vi "Handle MB Commands.vi"(4 "SP_CHAMBER":dbl, 6 "SP_DUT":dbl, 8 "error in (no error)":errorcluster, 10 "CMD REG":T1, 11 "Stand in":refnum<class "Stand.lvclass">) -> (0 "error out":errorcluster, 3 "Stand out":refnum<class "Stand.lvclass">)   [LabVIEW 2019, in "Stand.lvclass"]
uses:
  Stand.lvclass
  D:/GIT H4000/H4000/src/Device_class/Device.lvclass
  Modbus_class/CMD REG.ctl
  Stand.lvclass/Stand.ctl
  TypeDef/Mode.ctl
  Valve DIR.ctl
  Device_class/Device.lvclass/Device.ctl
  TypeDef/Direction.ctl
  TypeDef/State 44-1-2.ctl
  Valve Mode.ctl
  Device_class/GetFPGA.vi
  DoValve.vi
  Valve State Mode.vi
  DoValve.vi/e7d2c9dc-ba67-4685-b926-bcce34aa2778.vi
  DoValve.vi/628819af-fd07-4303-9780-3ddd467101db.vi
  Valve State Mode.vi/810e184e-eeb6-4027-a8ae-1422f3ce3d45.vi
  Valve State Mode.vi/57bd4a65-f3dc-44f5-8d68-677c2a197570.vi
  Valve State Mode.vi/03b2f9e4-fceb-4725-9b90-3fd10082a088.vi
  Valve State Mode.vi/2785bab5-dd59-4d13-b638-b9157202fa4a.vi
  Valve State Mode.vi/50faa4b8-a9b4-4cc6-ab66-55c42b424fcd.vi
  Valve State Mode.vi/c882c3fe-b7a7-4419-8f9b-6788aa23338b.vi
  Valve State Mode.vi/3d0d09bd-48e8-482f-b1e2-a36b2bb65234.vi
  Valve State Mode.vi/33d3f26a-dc4a-4f56-bf0a-61d04c5d7434.vi
  Valve State Mode.vi/52af9d47-24d1-4057-80bf-8d93bfb3d17d.vi
  Valve State Mode.vi/bbc9916c-129f-4456-975e-9c3ae3d5db66.vi
  Valve State Mode.vi/a6106d78-2bf9-477e-b655-d47fad07ddfe.vi
  Valve State Mode.vi/e2916439-03c6-4471-bb40-42242a636e27.vi
  Valve State Mode.vi/094228cb-a119-423c-9af8-5a16f059a318.vi
  Valve State Mode.vi/bf5ad1e6-a0ae-4579-ad74-ca8f304cb7cf.vi
  Valve State Mode.vi/eb4d2b76-f0f0-4e1d-bda0-609c5f37b4e7.vi
  Const All Valve.vi
  FPGA_API_class/FPGA API.lvclass
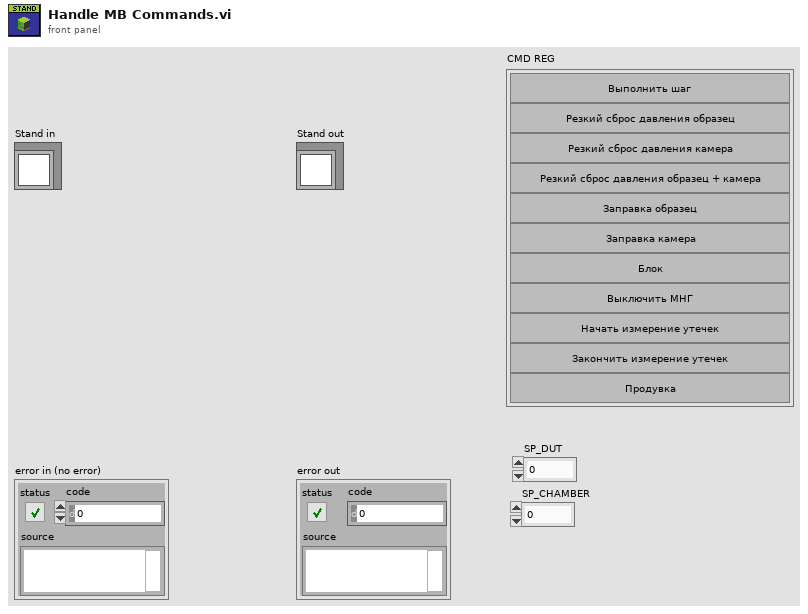
[diagram p1: front panel]
types:
  T1 = typedef "CMD REG.ctl" = cluster{"EXECUTE_SP":bool, "ALARM_PRESS_DOWN_DUT":bool, "ALARM_PRESS_DOWN_CHAMBER":bool, "ALARM_PRESS_DOWN_DUT_CHAMBER":bool, "FILING_DUT":bool, "FILING_CHAMBER":bool, "BLOCK":bool, "PUMP_STATION_OFF":bool, "Leak start":bool, "Leak stop":bool, "Drain":bool}
  T2 = typedef "Valve DIR.ctl" = enum16{"Air Valves: Open (DUT Filling)", "Air Valves: Open (Chamber Filling)", "Air Valves: Open (Pump Pressure DUT)", "Air Valves: Open (Pump Pressure Chamber)", "Air Valves: Open (Haskel Pressure DUT)", "Air Valves: Open (Haskel Pressure Chamber)", "Air Valves: Open (Slow Release DUT)", "Air Valves: Open (Slow Release Chamber)", "Air Valves: Open (Fast Release DUT)", "Air Valves: Open (Fast Release Chamber)", "Air Valves: Open (Emergency Release DUT and Chamber)", "Air Valves: Leak Hi (Chamber)", "Air Valves: Leak Hi (DUT)", "Air Valves: Backpressure (Chamber)", "Air Valves: Backpressure (DUT)", "Air Valves: Fully Closed", "Air Valves: Open 33.7"}
  T3 = typedef "Mode.ctl" = enum16{"IDLE", "FILLING", "EXECUTE_SP", "DRAIN"}
  T4 = typedef "Direction.ctl" = enum8{"DUT", "Chamber"}
  T5 = typedef "Valve Mode.ctl" = enum16{"Filling DUT", "Filling Chamber", "Pump Pressure DUT", "Pump Pressure Chamber", "Haskel Pressure DUT", "Haskel Pressure Chamber", "Slow Release DUT", "Slow Release Chamber", "Fast Release DUT", "Fast Release Chamber", "Fast Release DUT and Chamber", "Leak Pressure DUT", "Leak Pressure Chamber", "Back Pressure DUT", "Back Pressure Chamber", "Fully Closed", "Drain", "Block DUT", "Block Chamber", "filling dut down", "filling chamber down"}
  T6 = typedef "State 44-1-2.ctl" = enum16{"Init", "Idle", "Wait", "Open 44-1", "Open 44-2", "Close 44-1", "Close 44-2"}
  T7 = typedef "SP_TYPE.ctl" = enum16{"ERROR", "ZIRO", "BASE", "SP"}
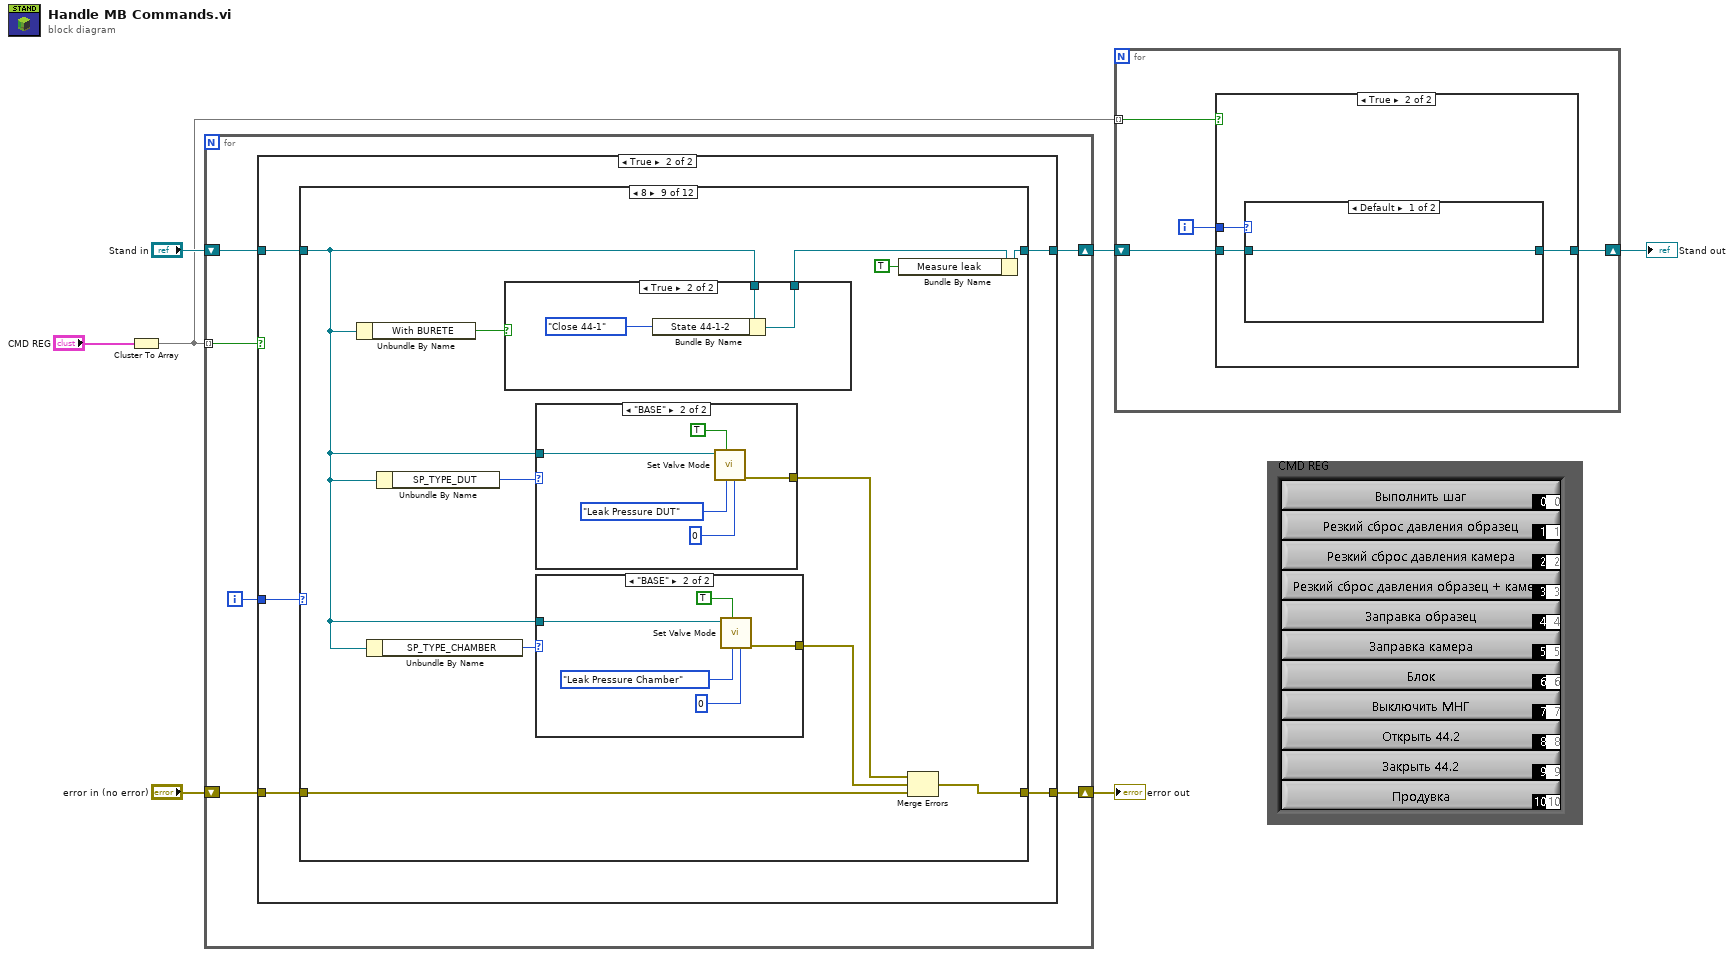
[diagram p0: block diagram]
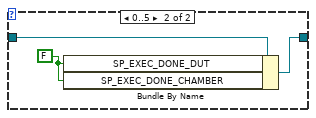
[diagram p3: hidden frame]
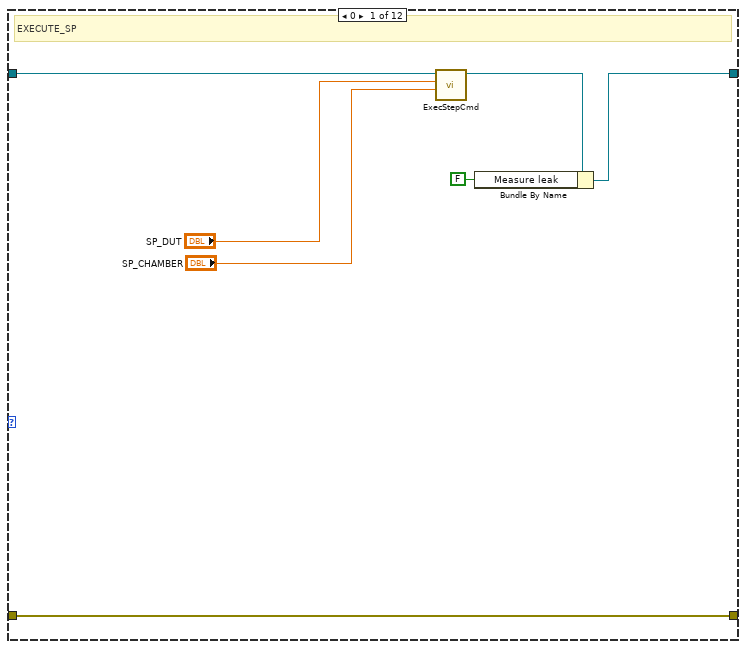
[diagram p5: hidden frame]
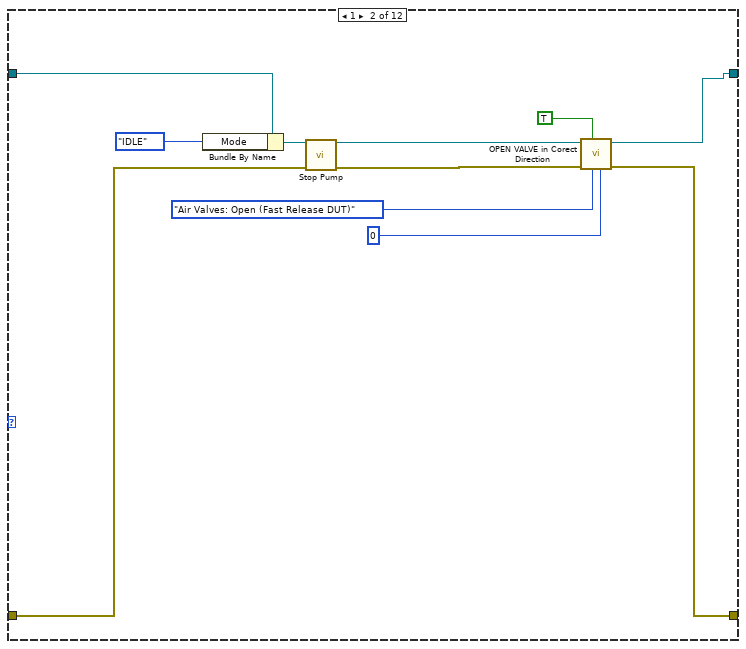
[diagram p6: hidden frame]
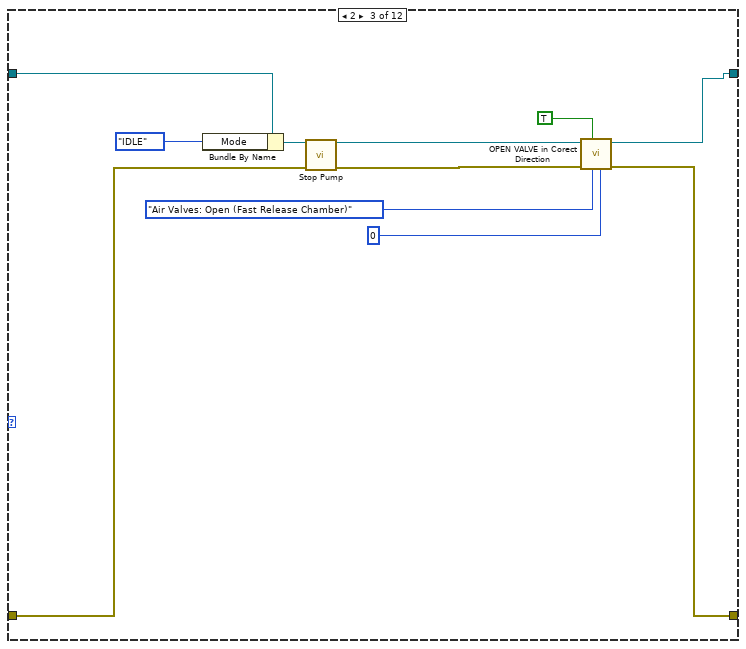
[diagram p7: hidden frame]
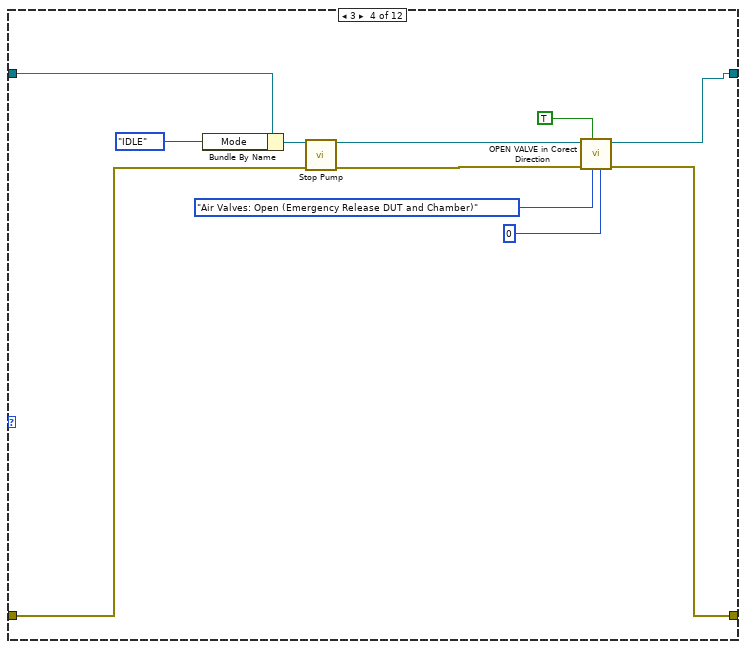
[diagram p8: hidden frame]
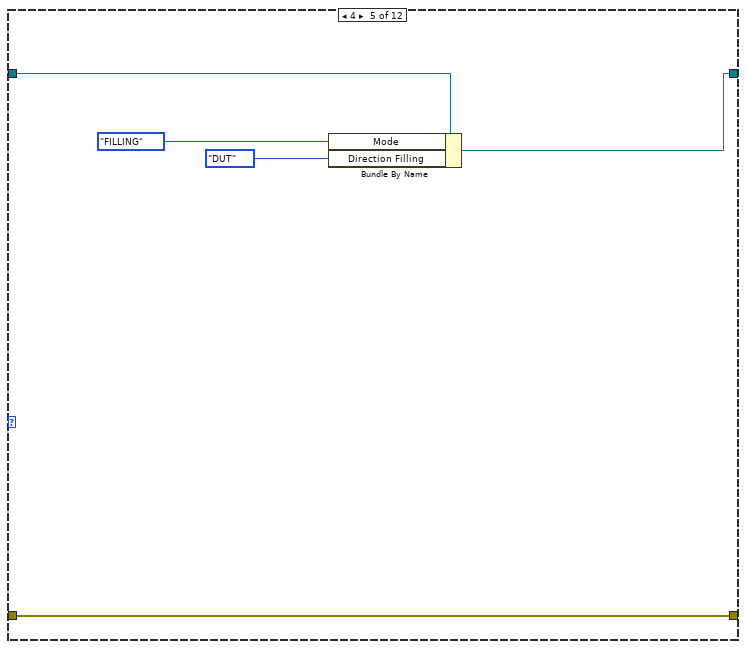
[diagram p9: hidden frame]
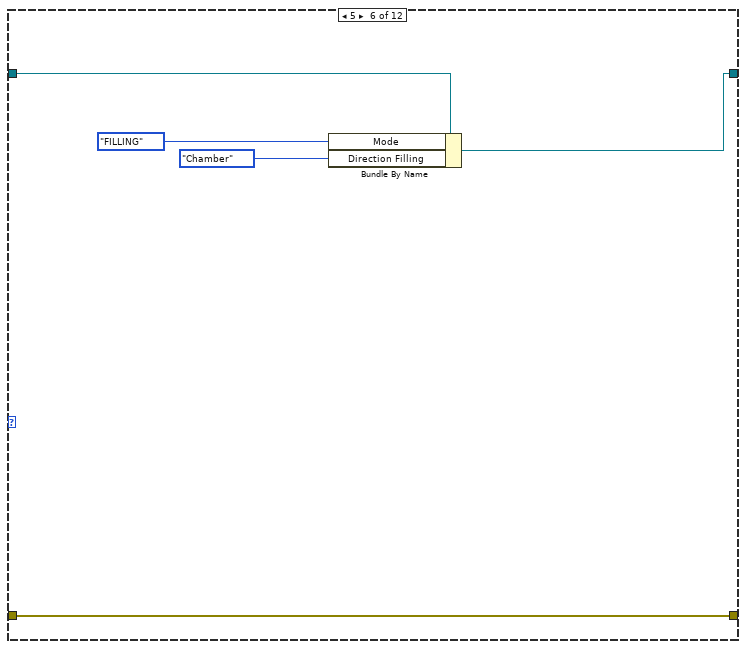
[diagram p10: hidden frame]
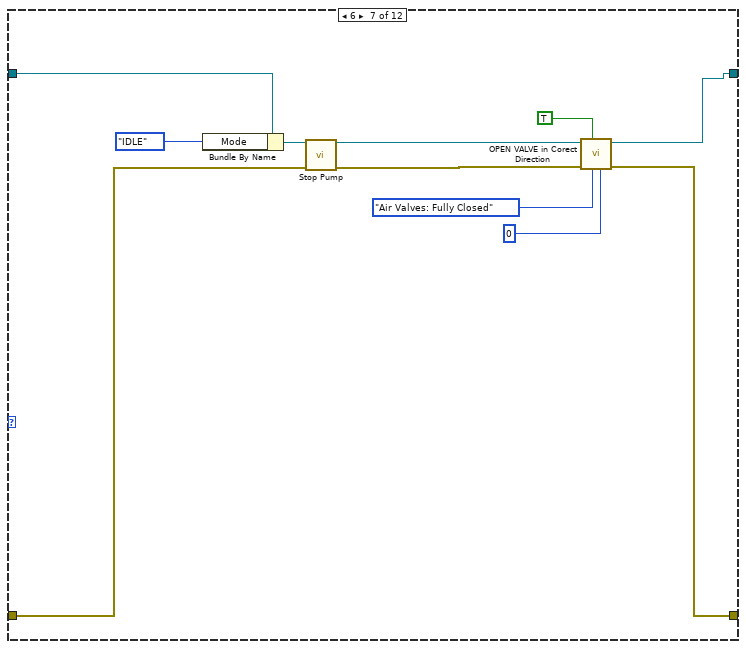
[diagram p11: hidden frame]
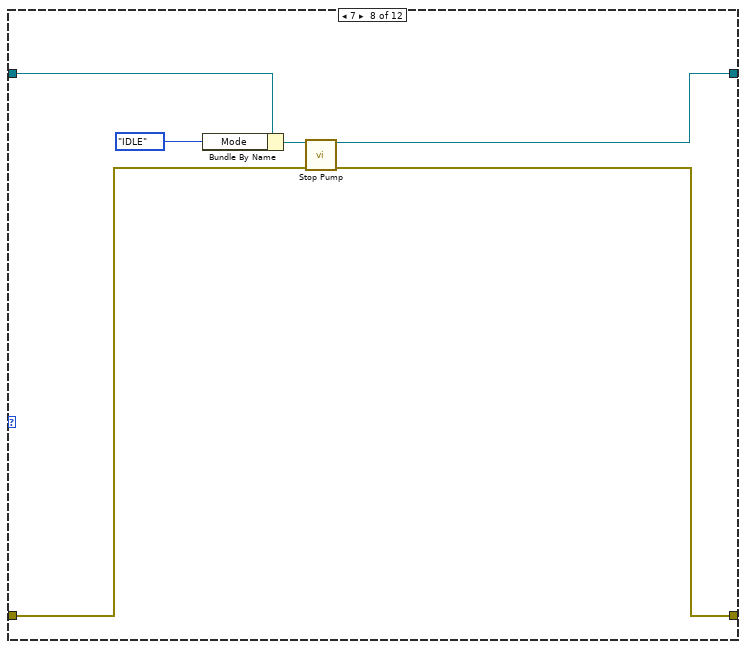
[diagram p12: hidden frame]
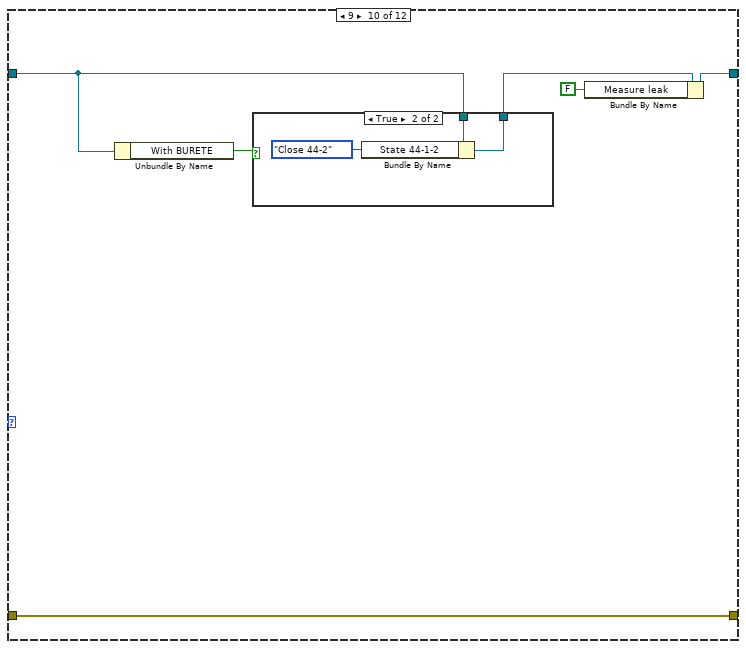
[diagram p16: hidden frame]
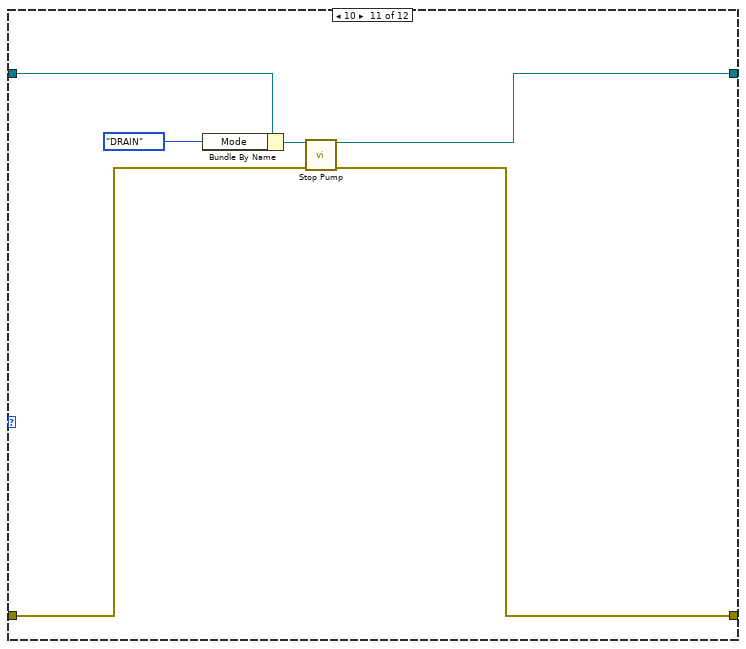
[diagram p18: hidden frame]
diagram:
  n1 = Cluster To Array(cluster="CMD REG") -> (array=w1:bool[])
  n2 = for {
    tunnel: w1 -> [w13] mode=indexing
    shift-right: [w8] -> w4
    shift-left: "Stand in" -> [w11]
    shift-right: [w10] -> w6
    shift-left: "error in (no error)" -> [w9]
    i -> [w12]
    n3 = case shown="True" w13 {
      tunnel: w12 -> [_ w17]
      tunnel: w11 -> [w15 w16]
      tunnel: [w14 w20] -> w10
      tunnel: w9 -> [w14 w19]
      tunnel: [w15 w18] -> w8
      frame False {
      }
      frame True {
        n4 = case shown="8" w17 {
          tunnel: w16 -> [w27 w31 w42 w53 w63 w68 w74 w83 w93 w116 w124 w130]
          tunnel: [w26 w28 w39 w50 w62 w67 w71 w84 w92 w118 w125 w129] -> w20
          tunnel: w19 -> [w26 w29 w40 w51 w62 w67 w72 w82 w98 w118 w123 w129]
          tunnel: [w21 w30 w41 w52 w64 w69 w73 w85 w89 w114 w126 w130] -> w18
          frame 0 {
            # "EXECUTE_SP"
            n5 = call "ExecStepCmd.vi"("SP_CHAMBER"="SP_CHAMBER", "SP_DUT"="SP_DUT", "Stand in"=w27) -> ("Stand out"=w22:refnum<class "Stand.lvclass">)  [unwired: 8 in]
            n6 = Bundle By Name(cluster=w22, "Measure leak"=FALSE ("Data.Measure leak")) -> (w21:refnum<class "Stand.lvclass">)
          }
          frame 1 {
            n7 = Bundle By Name(cluster=w31, "Mode"=Mode."IDLE" ("Data.Mode")) -> (w37:refnum<class "Stand.lvclass">)
            n8 = call "Stop Pump.vi"("reference in"=w37, "error in (no error)"=w29) -> ("reference out"=w36:refnum<class "Stand.lvclass">, "error out"=w35:errorcluster)  [unwired: 11 in, 1 out]
            n9 = call "OPEN VALVE in Corect Direction.vi"("time after close"=u32 0, "Valve DIR"=Valve_DIR."Air Valves: Open (Fast Release DUT)", "changed or first call?"=TRUE, "error in (no error)"=w35, "Stand in"=w36) -> ("error out"=w28:errorcluster, "Stand out"=w30:refnum<class "Stand.lvclass">)  [unwired: 4 in, 1 out]
          }
          frame 2 {
            n10 = Bundle By Name(cluster=w42, "Mode"=Mode."IDLE" ("Data.Mode")) -> (w48:refnum<class "Stand.lvclass">)
            n11 = call "Stop Pump.vi"("reference in"=w48, "error in (no error)"=w40) -> ("reference out"=w47:refnum<class "Stand.lvclass">, "error out"=w46:errorcluster)  [unwired: 11 in, 1 out]
            n12 = call "OPEN VALVE in Corect Direction.vi"("time after close"=u32 0, "Valve DIR"=Valve_DIR."Air Valves: Open (Fast Release Chamber)", "changed or first call?"=TRUE, "error in (no error)"=w46, "Stand in"=w47) -> ("error out"=w39:errorcluster, "Stand out"=w41:refnum<class "Stand.lvclass">)  [unwired: 4 in, 1 out]
          }
          frame 3 {
            n13 = Bundle By Name(cluster=w53, "Mode"=Mode."IDLE" ("Data.Mode")) -> (w59:refnum<class "Stand.lvclass">)
            n14 = call "Stop Pump.vi"("reference in"=w59, "error in (no error)"=w51) -> ("reference out"=w58:refnum<class "Stand.lvclass">, "error out"=w57:errorcluster)  [unwired: 11 in, 1 out]
            n15 = call "OPEN VALVE in Corect Direction.vi"("time after close"=u32 0, "Valve DIR"=Valve_DIR."Air Valves: Open (Emergency Release DUT and Chamber)", "changed or first call?"=TRUE, "error in (no error)"=w57, "Stand in"=w58) -> ("error out"=w50:errorcluster, "Stand out"=w52:refnum<class "Stand.lvclass">)  [unwired: 4 in, 1 out]
          }
          frame 4 {
            n16 = Bundle By Name(cluster=w63, "Mode"=Mode."FILLING" ("Data.Mode"), "Direction Filling"=Direction."DUT" ("Data.Direction Filling")) -> (w64:refnum<class "Stand.lvclass">)
          }
          frame 5 {
            n17 = Bundle By Name(cluster=w68, "Mode"=Mode."FILLING" ("Data.Mode"), "Direction Filling"=Direction."Chamber" ("Data.Direction Filling")) -> (w69:refnum<class "Stand.lvclass">)
          }
          frame 6 {
            n18 = Bundle By Name(cluster=w74, "Mode"=Mode."IDLE" ("Data.Mode")) -> (w80:refnum<class "Stand.lvclass">)
            n19 = call "Stop Pump.vi"("reference in"=w80, "error in (no error)"=w72) -> ("reference out"=w79:refnum<class "Stand.lvclass">, "error out"=w78:errorcluster)  [unwired: 11 in, 1 out]
            n20 = call "OPEN VALVE in Corect Direction.vi"("time after close"=u32 0, "Valve DIR"=Valve_DIR."Air Valves: Fully Closed", "changed or first call?"=TRUE, "error in (no error)"=w78, "Stand in"=w79) -> ("error out"=w71:errorcluster, "Stand out"=w73:refnum<class "Stand.lvclass">)  [unwired: 4 in, 1 out]
          }
          frame 7 {
            n21 = Bundle By Name(cluster=w83, "Mode"=Mode."IDLE" ("Data.Mode")) -> (w86:refnum<class "Stand.lvclass">)
            n22 = call "Stop Pump.vi"("reference in"=w86, "error in (no error)"=w82) -> ("reference out"=w85:refnum<class "Stand.lvclass">, "error out"=w84:errorcluster)  [unwired: 11 in, 1 out]
          }
          frame 8 {
            n23 = Unbundle By Name(w93) -> ("With BURETE"=w96:bool)
            n24 = Unbundle By Name(w93) -> ("SP_TYPE_CHAMBER"=w94:T7)
            n25 = Unbundle By Name(w93) -> ("SP_TYPE_DUT"=w95:T7)
            n26 = case shown="True" w96 {
              tunnel: [w109 w112] -> w97
              tunnel: w93 -> [w109 w110]
              frame False {
              }
              frame True {
                n27 = Bundle By Name(cluster=w110, "State 44-1-2"=State_44-1-2."Close 44-1" ("Data.State 44-1-2")) -> (w112:refnum<class "Stand.lvclass">)
              }
            }
            n28 = case shown="\"BASE\"" w95 {
              tunnel: w93 -> [_ w106]
              tunnel: [_ w105] -> w90
              frame Default {
              }
              frame "BASE" {
                n29 = call "Set Valve Mode.vi"("time after close"=u32 0, "Valve DIR"=Valve_Mode."Leak Pressure DUT", "init"=TRUE, "Stand in"=w106) -> ("error out"=w105:errorcluster)  [unwired: 6 in, 1 out]
              }
            }
            n30 = case shown="\"BASE\"" w94 {
              tunnel: w93 -> [_ w101]
              tunnel: [_ w100] -> w91
              frame Default {
              }
              frame "BASE" {
                n31 = call "Set Valve Mode.vi"("time after close"=u32 0, "Valve DIR"=Valve_Mode."Leak Pressure Chamber", "init"=TRUE, "Stand in"=w101) -> ("error out"=w100:errorcluster)  [unwired: 6 in, 1 out]
              }
            }
            n32 = Bundle By Name(cluster=w97, "Measure leak"=TRUE ("Data.Measure leak")) -> (w89:refnum<class "Stand.lvclass">)
            n33 = Merge Errors(w90, w91, w98) -> (w92:errorcluster)
          }
          frame 9 {
            n34 = Unbundle By Name(w116) -> ("With BURETE"=w115:bool)
            n35 = case shown="True" w115 {
              tunnel: [w119 w122] -> w117
              tunnel: w116 -> [w119 w120]
              frame False {
              }
              frame True {
                n36 = Bundle By Name(cluster=w120, "State 44-1-2"=State_44-1-2."Close 44-2" ("Data.State 44-1-2")) -> (w122:refnum<class "Stand.lvclass">)
              }
            }
            n37 = Bundle By Name(cluster=w117, "Measure leak"=FALSE ("Data.Measure leak")) -> (w114:refnum<class "Stand.lvclass">)
          }
          frame 10 {
            n38 = Bundle By Name(cluster=w124, "Mode"=Mode."DRAIN" ("Data.Mode")) -> (w127:refnum<class "Stand.lvclass">)
            n39 = call "Stop Pump.vi"("reference in"=w127, "error in (no error)"=w123) -> ("reference out"=w126:refnum<class "Stand.lvclass">, "error out"=w125:errorcluster)  [unwired: 11 in, 1 out]
          }
          frame Default {
          }
        }
      }
    }
  }
  "error out" <- w6
  n40 = for {
    shift-right: [w132] -> w3
    shift-left: w4 -> [w133]
    tunnel: w1 -> [w134] mode=indexing
    i -> [w131]
    n41 = case shown="True" w134 {
      tunnel: w133 -> [w135 w136]
      tunnel: [w135 w137] -> w132
      tunnel: w131 -> [_ w138]
      frame False {
      }
      frame True {
        n42 = case shown="Default" w138 {
          tunnel: [w139 w140] -> w137
          tunnel: w136 -> [w139 w141]
          frame Default {
          }
          frame 0..5 {
            w142 = FALSE ("Data.STS.SP_EXEC_DONE_DUT")
            n43 = Bundle By Name(cluster=w141, "SP_EXEC_DONE_DUT"=w142, "SP_EXEC_DONE_CHAMBER"=w142) -> (w140:refnum<class "Stand.lvclass">)
          }
        }
      }
    }
  }
  "Stand out" <- w3
